vi "SpecAn Ref Level Read.vi"(0 "VISA In":refnum<visa-resource-name>, 5 "Error In":errorcluster) -> (12 "Ref Level (dBm)":dbl, 14 "VISA Out":refnum<visa-resource-name>, 19 "Error Out":errorcluster)   [LabVIEW 2015]
uses:
  Controls/FGV Action SpecAn Model.ctl
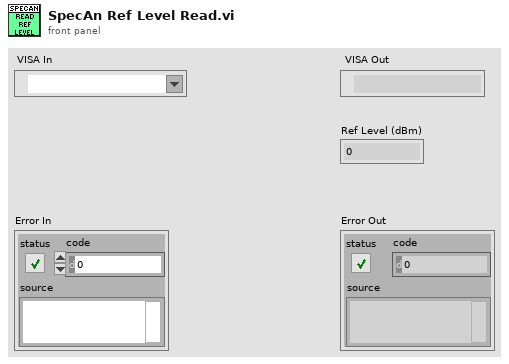
[diagram p1: front panel]
types:
  T1 = typedef "FGV Action SpecAn Model.ctl" = enum16{"Get", "Set"}
  T2 = typedef "SpecAn Model.ctl" = enum16{"E4440", "N9030"}
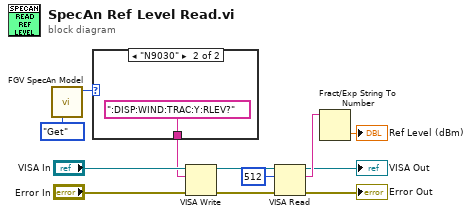
[diagram p0: block diagram]
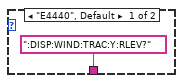
[diagram p2: hidden frame]
diagram:
  n1 = call "FGV SpecAn Model.vi"("Action"=FGV_Action_SpecAn_Model."Get") -> ("SA Model"=w9:T2)  [unwired: 6 in, 1 out]
  n2 = case shown="\"N9030\"" w9 {
    tunnel: [":DISP:WIND:TRAC:Y:RLEV?" ("format string") ":DISP:WIND:TRAC:Y:RLEV?" ("format string")] -> w8
    frame "E4440", Default {
    }
    frame "N9030" {
    }
  }
  n3 = VISA Write(VISA resource name="VISA In", write buffer=w8, error in (no error)="Error In") -> (VISA resource name out=w2:refnum<visa-resource-name>, error out=w5:errorcluster)  [unwired: 1 out]
  n4 = VISA Read(VISA resource name=w2, byte count=u32 512, error in (no error)=w5) -> (VISA resource name out=→"VISA Out":refnum<visa-resource-name>, read buffer=w6:string, error out=→"Error Out":errorcluster)  [unwired: 1 out]
  n5 = Fract/Exp String To Number(string=w6) -> (number=→"Ref Level (dBm)":dbl)  [unwired: 3 in, 1 out]
